vi "Write Formatters.vi"(8 "error in (no error)":errorcluster, 10 "Formatters":refnum<class "Formatter.lvclass">[](array[class]), 11 "Report in":refnum<class "Report.lvclass">) -> (0 "error out":errorcluster, 3 "Report out":refnum<class "Report.lvclass">)   [LabVIEW 2015, in "Report.lvclass"]
uses:
  Report.lvclass
  Report Formatters/Base Class/Execution/Formatter.lvclass
  Report.lvclass/Report.ctl
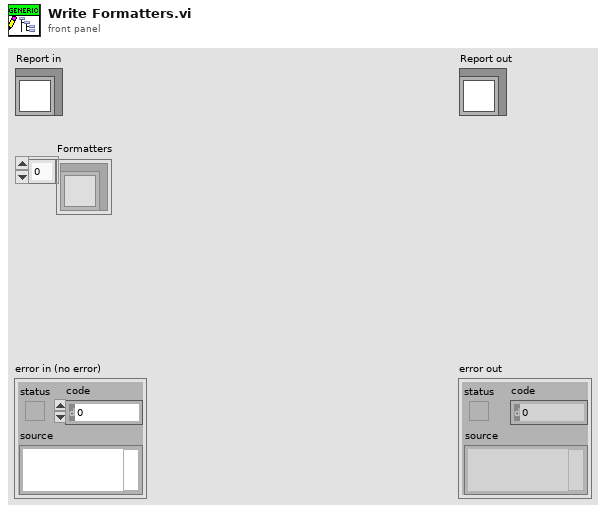
[diagram p1: front panel]
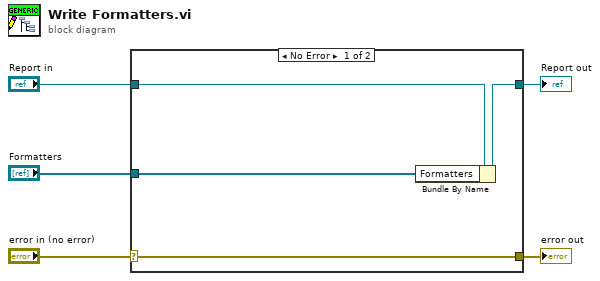
[diagram p0: block diagram]
diagram:
  n1 = case shown="No Error" "error in (no error)" {
    selector: "error in (no error)" -> [w9 w10]
    tunnel: [w9 w10] -> w4
    tunnel: [w7 w11] -> w2
    tunnel: "Report in" -> [w8 w11]
    tunnel: "Formatters" -> [w6 _]
    frame No Error {
      n2 = Bundle By Name(cluster=w8, "Formatters"=w6) -> (w7:refnum<class "Report.lvclass">)
    }
    frame Error {
    }
  }
  "error out" <- w4
  "Report out" <- w2
